vi "Create (Array).vi"(10 "error in (no error)":errorcluster, 11 "Bindings":string[](array[string])) -> (2 "error out":errorcluster, 3 "IP Resolver":refnum<class "IP Resolver.lvclass">)   [LabVIEW 2020, in "Vecto.lvlib" / "IP Resolver.lvclass"]
uses:
  IP Resolver.lvclass
  Bind Info.ctl
  Address Type.ctl
  IP Resolver.lvclass/IP Resolver.ctl
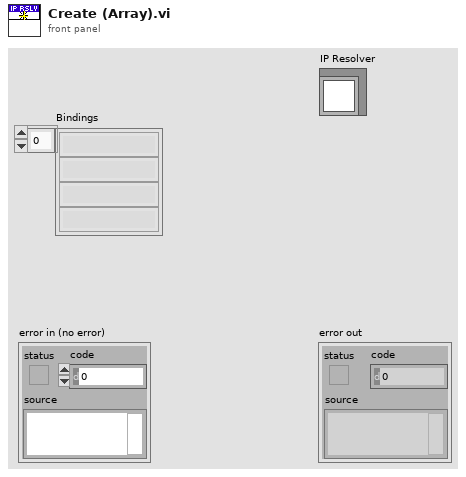
[diagram p1: front panel]
types:
  T1 = typedef "Vecto.lvlib/IP Resolver.lvclass/Address Type.ctl" = enum16{"Unknown", "Specific", "Subnet", "Any"}
  T2 = typedef "Vecto.lvlib/IP Resolver.lvclass/Bind Info.ctl" = cluster{"Type":T1, "Binding":string, "Subnet Bits":i32}
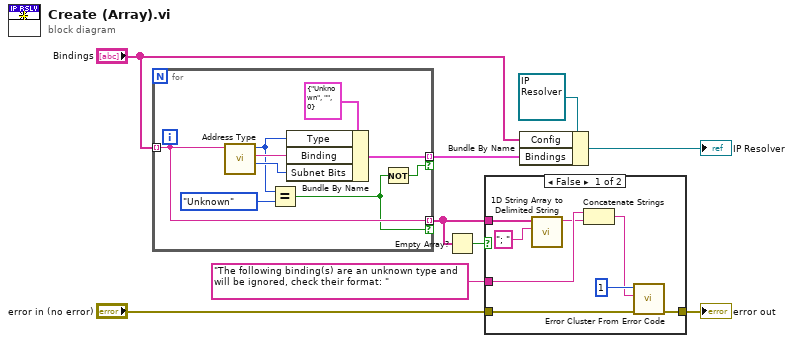
[diagram p0: block diagram]
diagram:
  n1 = for {
    tunnel: "Bindings" -> [w11] mode=indexing
    tunnel: [w15] -> w7 mode=indexing if=w12
    tunnel: [w11] -> w5 mode=indexing if=w10
    n2 = call "Address Type.vi"("Address In"=w11) -> ("Subnet Bits"=w16:i32, "Address"=w17:string, "Address Type"=w14:T1)  [unwired: 8 in]
    n3 = Equal?(x=w14, y=Address_Type."Unknown") -> (x = y?=w10:bool)
    n4 = Bundle By Name(cluster=T2 {"Type"=enum."Unknown", "Binding"="", "Subnet Bits"=0} ("Bind Info"), "Type"=w14, "Binding"=w17, "Subnet Bits"=w16) -> (w15:T2)
    n5 = Not(x=w10) -> (.not. x?=w12:bool)
  }
  n6 = Empty Array?(array=w5) -> (empty?=w4:bool)
  n7 = case shown="False" w4 {
    tunnel: w5 -> [w26 _]
    tunnel: "error in (no error)" -> [w22 w27]
    tunnel: [w19 w27] -> w2
    tunnel: "The following binding(s) are an unknown type and will be ignored, check their format: " -> [w24 _]
    frame False {
      n8 = call <vilib>:"1D String Array to Delimited String.vi"("delimiter"="; ", "string array"=w26) -> ("delimited string"=w23:string)  [unwired: 9 in]
      n9 = Concatenate Strings(w24, w23) -> (w20:string)
      n10 = call <vilib>:"Error Cluster From Error Code.vi"("error in (no error)"=w22, "error message (\"\")"=w20, "error code (0)"=1) -> ("error out"=w19:errorcluster)  [unwired: 6 in]
    }
    frame True {
    }
  }
  "error out" <- w2
  n11 = Bundle By Name(cluster=refnum<class "IP Resolver.lvclass"> refnum ("IP Resolver in"), "Config"="Bindings", "Bindings"=w7) -> (→"IP Resolver":refnum<class "IP Resolver.lvclass">)
